vi "Abort Python Script.vi"(7 "Server Alias":string, 8 "error in (no error)":errorcluster, 11 "Script ID to Abort":i64) -> (0 "error out":errorcluster)   [LabVIEW 2013, in "TS.lvlib"]
doc: "This VI aborts the script with Script_ID to Abort. It's sending a particular message to Python."
uses:
  TS.lvlib
  LabVIEW Python Connector Message.ctl
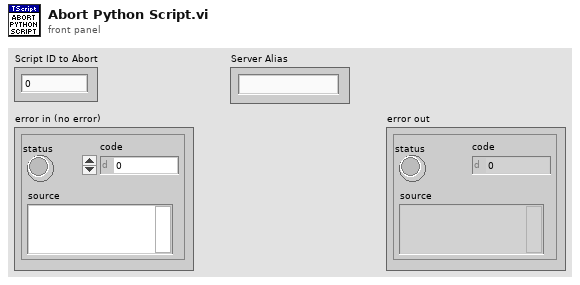
[diagram p1: front panel]
types:
  T1 = typedef "TS.lvlib/LabVIEW Python Connector Message.ctl" = cluster{"Command":string, "Data":string[], "Script ID":i64, "LabVIEW Server ID":string, "Python Message ID":i32}
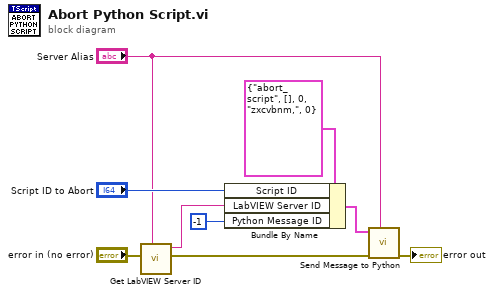
[diagram p0: block diagram]
diagram:
  n1 = call "Get LabVIEW Server ID.vi"("Server Alias"="Server Alias", "Error In"="error in (no error)") -> ("Error Out"=w2:errorcluster, "LabVIEW Server ID"=w4:string)  [unwired: 8 in]
  n2 = Bundle By Name(cluster=T1 {"Command"="abort_script", "Data"=[], "Script ID"=0, "LabVIEW Server ID"="zxcvbnm,", "Python Message ID"=0} ("Message"), "Script ID"="Script ID to Abort", "LabVIEW Server ID"=w4, "Python Message ID"=-1) -> (w7:T1)
  n3 = call "Send Message to Python.vi"("Server Alias"="Server Alias", "error in (no error)"=w2, "Message"=w7) -> ("error out"=→"error out":errorcluster)  [unwired: 8 in]
